vi "onHttpHead.vi"(8 "error in":errorcluster, 10 "httpRequest":refnum<class "httpRequest.lvclass">, 11 "advanced-http-client in":refnum<class "advanced-http-client.lvclass">) -> (0 "error out":errorcluster, 2 "httpResponse":refnum<class "httpResponse.lvclass">, 3 "advanced-http-client out":refnum<class "advanced-http-client.lvclass">)   [LabVIEW 2020, in "HttpClient.NiAdvanced.lvlib" / "advanced-http-client.lvclass"]
uses:
  advanced-http-client.lvclass
  advanced-http-client.lvclass/advanced-http-client.ctl
  <vilib>/NI/Advanced HTTP Client/Session.lvclass
  http-client-pkg/httpRequest/httpRequest.lvclass
  http-client-pkg/httpResponse/httpResponse.lvclass
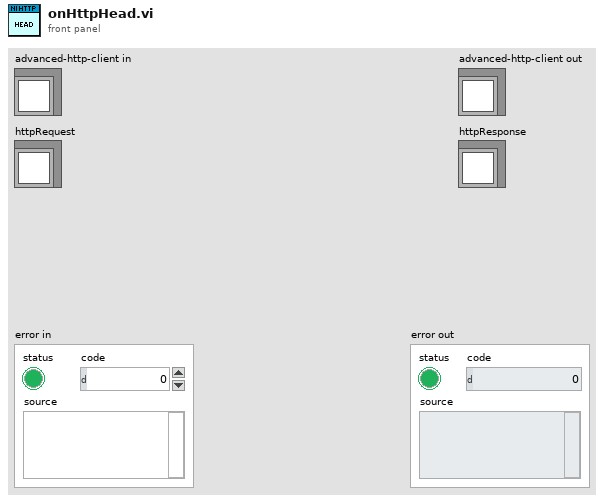
[diagram p1: front panel]
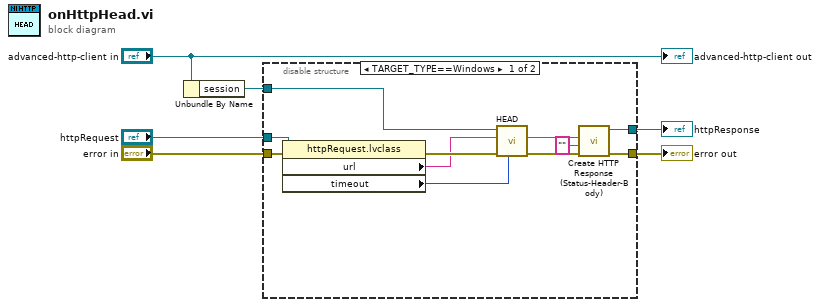
[diagram p0: block diagram]
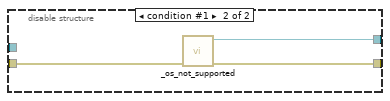
[diagram p2: hidden frame]
diagram:
  n1 = Unbundle By Name("advanced-http-client in") -> ("session"=w2:refnum<class "Session.lvclass">)
  n2 = disable-structure shown="TARGET_TYPE==Windows" {
    disable-tunnel: [w10 w19] -> w6
    disable-tunnel: "error in" -> [w14 w20]
    disable-tunnel: "httpRequest" -> [w16 _]
    disable-tunnel: w2 -> [w17 _]
    disable-tunnel: [w9 w18] -> w1
    frame condition #0 (active) {
      n3 = property class="httpRequest.lvclass"(reference=w16, error in=w14) -> (error out=w15:errorcluster, "url"=w13:string, "timeout"=w12:i32)  [unwired: 1 out]
      n4 = call <vilib>:"HEAD.vi"("timeout"=w12, "error in"=w15, "url"=w13, "session in"=w17) -> ("error out"=w11:errorcluster, "headers"=w8:string)  [unwired: 4 in, 2 out]
      n5 = call "Create HTTP Response (Status-Header-Body).vi"("error in"=w11, "body"="", "Headers w/ status line(s)"=w8) -> ("error out"=w10:errorcluster, "httpResponse out"=w9:refnum<class "httpResponse.lvclass">)  [unwired: 7 in]
    }
    frame condition #1 {
      n6 = call "_os_not_supported.vi"("error in (no error)"=w20) -> ("error out"=w19:errorcluster, "httpResponse"=w18:refnum<class "httpResponse.lvclass">)  [unwired: 9 in]
    }
  }
  "error out" <- w6
  "httpResponse" <- w1
  "advanced-http-client out" <- "advanced-http-client in"
